vi "tls get error string.vi"(8 "error in":errorcluster, 11 "tls context":u64) -> (0 "error out":errorcluster, 3 "error string":string)   [LabVIEW 2016, in "lv tls dll.lvlib"]
uses:
  lv tls dll.lvlib
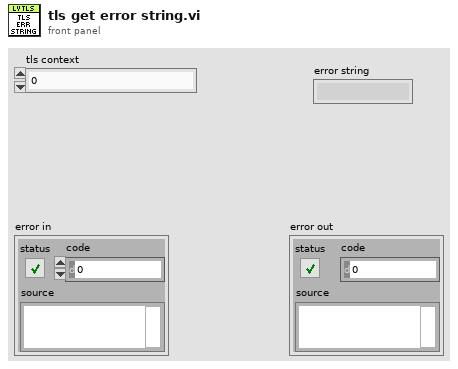
[diagram p1: front panel]
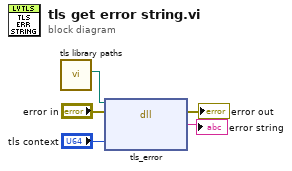
[diagram p0: block diagram]
diagram:
  n1 = call "tls library paths.vi"() -> ("libtls"=w5:path)  [unwired: 8 in, 3 out]
  n2 = dll-call lib="C:/Users/IEUser/Desktop/tlssimple/libtls-15.dll" fn="tls_error"(path in=w5, error in="error in", "context"="tls context") -> (error out=→"error out":errorcluster, "err"=→"error string":string)  [unwired: 2 in, 1 out]
